vi "Prepare Data.vi"(11 "Data Cluster":T1) -> (2 "WiBCI 16T Data":T2 {"Reg Map"."ADS2" format="%x"; "Reg Map"."ADS1" format="%x"}, 3 "Module Data cluster out":T1)   [LabVIEW 2019, in "DemoData Generator.lvlib"]
uses:
  DemoData Generator.lvlib
  Acquisition/WiBCI16T_Data.ctl
  Acquisition/WiBCI16T_Status.ctl
  Acquisition/Reg_Map.ctl
  Module Data--cluster.ctl
  <vilib>/Utility/file.llb/Read Delimited Spreadsheet (DBL).vi
  Acquisition/Acquisition.lvlib
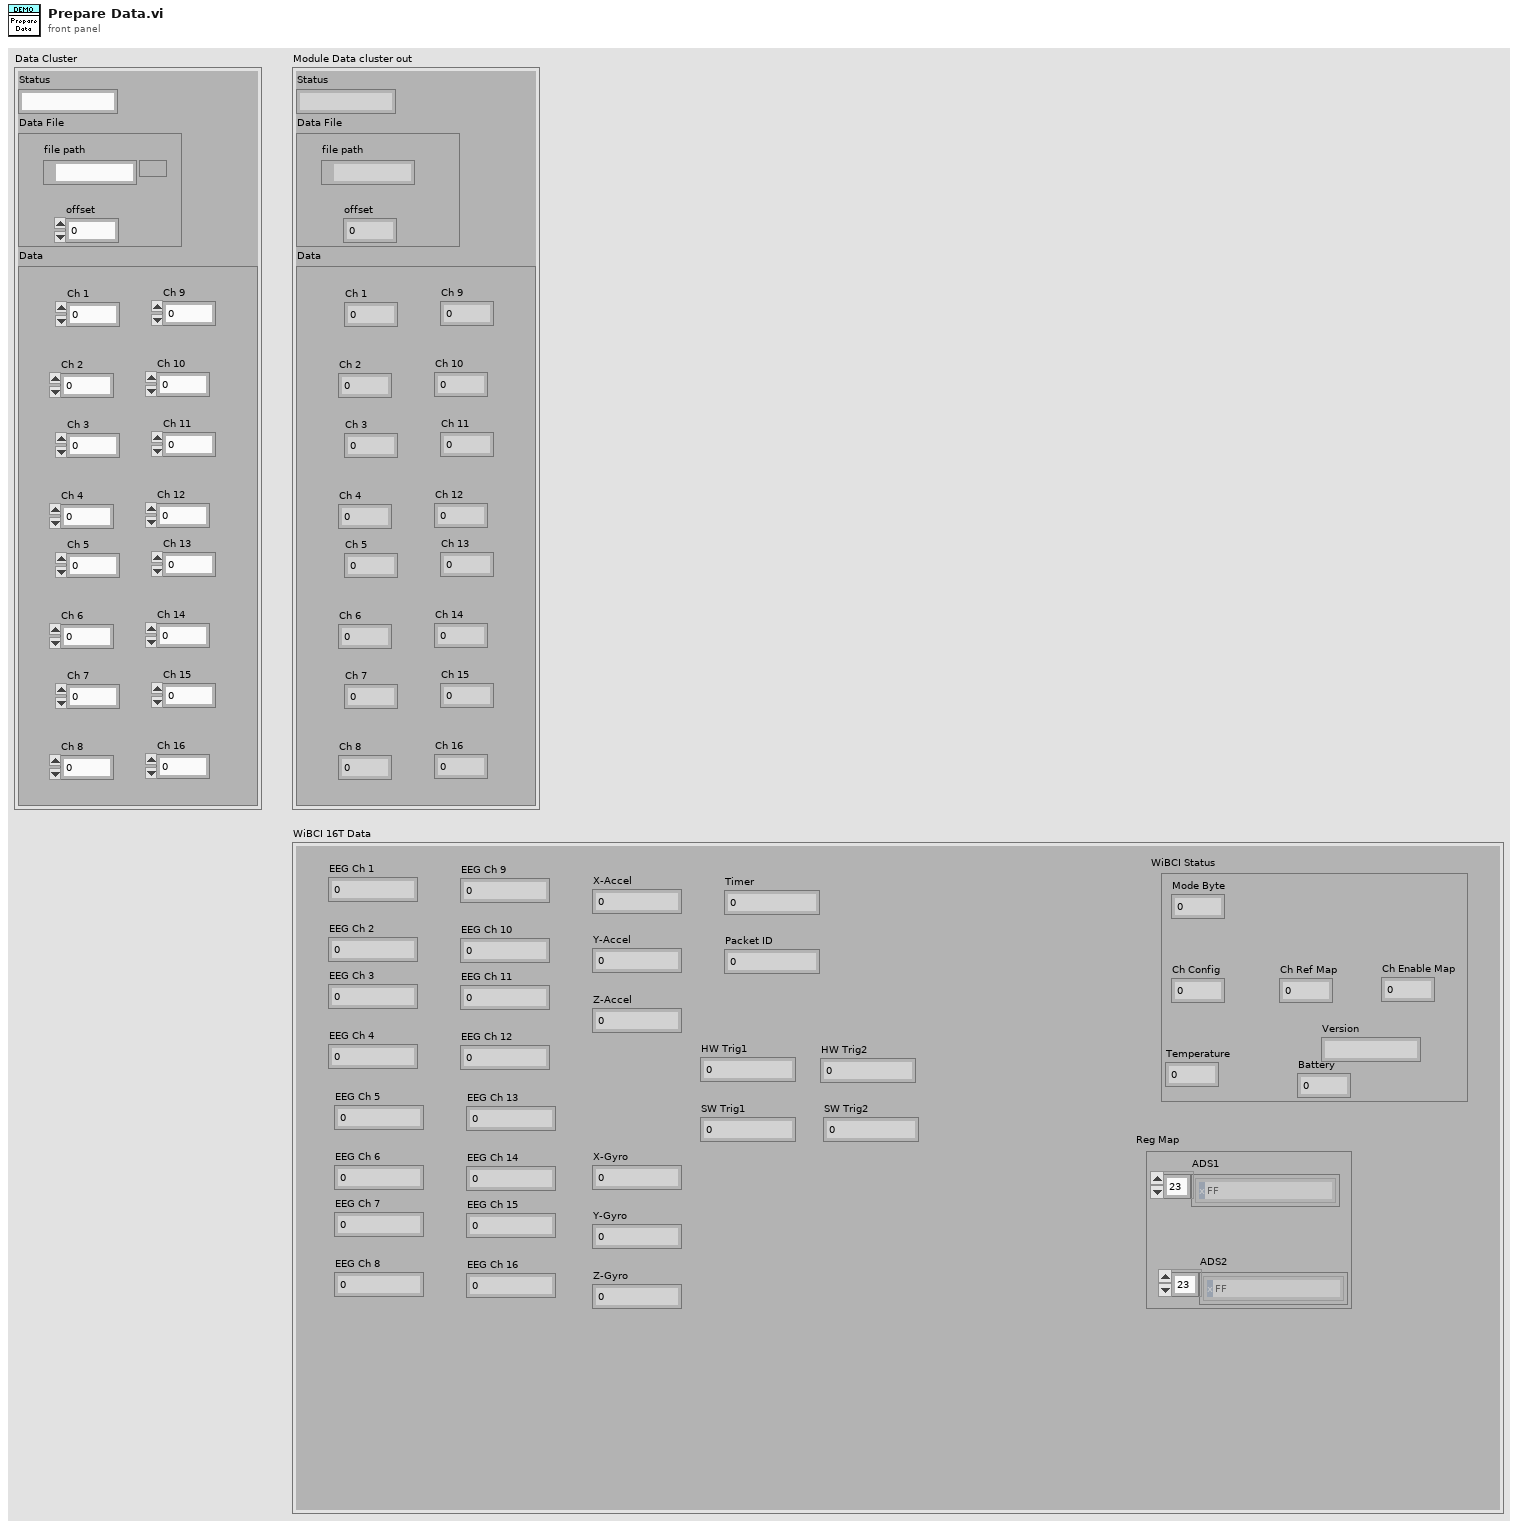
[diagram p1: front panel]
types:
  T1 = typedef "DemoData Generator.lvlib/Module Data--cluster.ctl" = cluster{"Status":string, "Data File":cluster{"file path":path, "offset":i32}, "Data":cluster{"Ch 1":dbl, "Ch 2":dbl, "Ch 3":dbl, "Ch 4":dbl, "Ch 5":dbl, "Ch 6":dbl, "Ch 7":dbl, "Ch 8":dbl, "Ch 9":dbl, "Ch 10":dbl, "Ch 11":dbl, "Ch 12":dbl, "Ch 13":dbl, "Ch 14":dbl, "Ch 15":dbl, "Ch 16":dbl}}
  T2 = typedef "Acquisition.lvlib/WiBCI16T_Data.ctl" = cluster{"EEG Ch 1":dbl, "EEG Ch 2":dbl, "EEG Ch 3":dbl, "EEG Ch 4":dbl, "EEG Ch 5":dbl, "EEG Ch 6":dbl, "EEG Ch 7":dbl, "EEG Ch 8":dbl, "EEG Ch 9":dbl, "EEG Ch 10":dbl, "EEG Ch 11":dbl, "EEG Ch 12":dbl, "EEG Ch 13":dbl, "EEG Ch 14":dbl, "EEG Ch 15":dbl, "EEG Ch 16":dbl, "X-Accel":i16, "Y-Accel":i16, "Z-Accel":i16, "X-Gyro":i16, "Y-Gyro":i16, "Z-Gyro":i16, "Timer":u32, "Packet ID":u32, "HW Trig1":u8, "SW Trig1":i8, "HW Trig2":u8, "SW Trig2":i8, "WiBCI Status":T3, "Reg Map":T4}
  T3 = typedef "Acquisition.lvlib/WiBCI16T_Status.ctl" = cluster{"Mode Byte":u8, "Ch Config":u8, "Ch Ref Map":u16, "Ch Enable Map":u16, "Temperature":sgl, "Battery":u8, "Version":string}
  T4 = typedef "Acquisition.lvlib/Reg_Map.ctl" = cluster{"ADS1":u8[], "ADS2":u8[]}
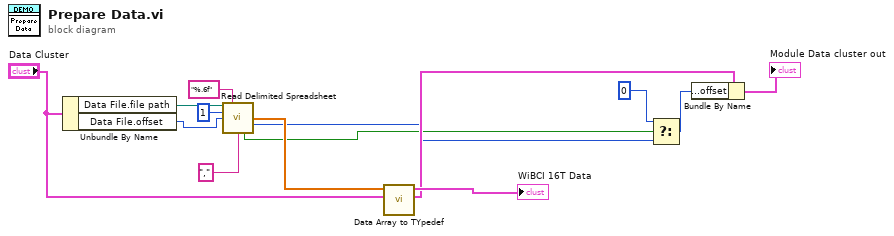
[diagram p0: block diagram]
diagram:
  n1 = Unbundle By Name("Data Cluster") -> ("Data File.file path"=w1:path, "Data File.offset"=w4:i32)
  n2 = call-poly <vilib>:"Read Delimited Spreadsheet.vi"("file path (dialog if empty)"=w1, "format (%.3f)"="%.6f", "number of rows (all:-1)"=1, "start of read offset (chars.:0)"=w4, "delimiter (\\t)"=",") -> ("first row"=w11:dbl[], "mark after read (chars.)"=w9:i32, "EOF?"=w7:bool)  [unwired: 5 in, 3 out]
  n3 = call "Data Array to TYpedef.vi"("Module Data Cluster"="Data Cluster", "first row"=w11) -> ("Module Data cluster out"=w13:T1, "WiBCI 16T Data"=→"WiBCI 16T Data":T2)  [unwired: 8 in]
  n4 = Select(t=0 ("Data File.offset"), s=w7, f=w9) -> (s? t:f=w10:i32)
  n5 = Bundle By Name(cluster=w13, "Data File.offset"=w10) -> (→"Module Data cluster out":T1)
